vi "quantizzatore.vi"(8 "Segnale input":waveform(dbl), 9 "B (# Bits)":dbl, 10 "Vfs":dbl, 11 "Tipo (bipolare = true)":bool) -> (0 "Livelli":dbl[](array[numeric]), 1 "Segnale quantizzato":waveform(dbl), 2 "2^B":dbl, 3 "Q":dbl)   [LabVIEW 2009]
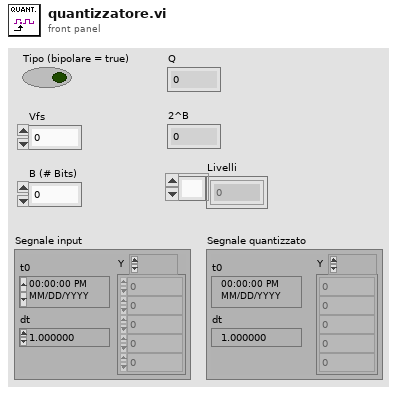
[diagram p1: front panel]
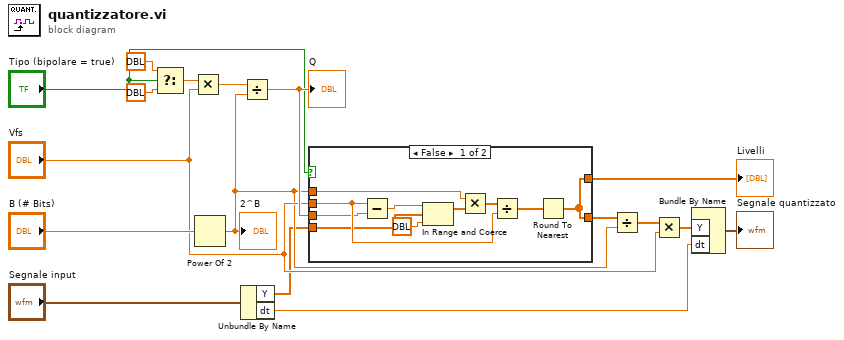
[diagram p0: block diagram]
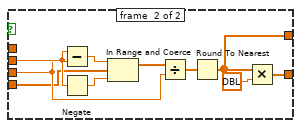
[diagram p2: hidden frame]
diagram:
  n1 = Select(t=dbl ?, s="Tipo (bipolare = true)", f=dbl ?) -> (s? t:f=w13:dbl)
  n2 = Multiply(x=w13, y="Vfs") -> (x*y=w14:dbl)
  n3 = Power Of 2(x="B (# Bits)") -> (2^x=w8:dbl)
  "2^B" <- w8
  n4 = Unbundle By Name("Segnale input") -> ("Y"=w6:dbl[], "dt"=w4:dbl)
  n5 = Divide(x=w14, y=w8) -> (x/y=w17:dbl)
  "Q" <- w17
  n6 = case shown="False" "Tipo (bipolare = true)" {
    tunnel: w6 -> [w24 w32]
    tunnel: [w18 w28] -> w2
    tunnel: "Vfs" -> [w27 w37]
    tunnel: w8 -> [w21 _]
    tunnel: w17 -> [w26 w36]
    tunnel: [w18 w30] -> w1
    frame #0 {
      n7 = Subtract(x=w27, y=w26) -> (x-y=w23:dbl)
      n8 = In Range and Coerce(upper limit=w23, x=w24, lower limit=dbl ?) -> (coerced(x)=w22:dbl[])  [unwired: 1 out]
      n9 = Multiply(x=w21, y=w22) -> (x*y=w20:dbl[])
      n10 = Divide(x=w20, y=w27) -> (x/y=w19:dbl[])
      n11 = Round To Nearest(number=w19) -> (nearest integer value=w18:dbl[])
    }
    frame #1 {
      n12 = Subtract(x=w37, y=w36) -> (x-y=w31:dbl)
      n13 = Negate(x=w37) -> (-x=w33:dbl)
      n14 = In Range and Coerce(upper limit=w31, x=w32, lower limit=w33) -> (coerced(x)=w34:dbl[])  [unwired: 1 out]
      n15 = Divide(x=w34, y=w36) -> (x/y=w35:dbl[])
      n16 = Round To Nearest(number=w35) -> (nearest integer value=w30:dbl[])
      n17 = Multiply(x=w30, y=dbl ?) -> (x*y=w28:dbl[])
    }
  }
  "Livelli" <- w1
  n18 = Divide(x=w2, y=w8) -> (x/y=w16:dbl[])
  n19 = Multiply(x=w16, y="Vfs") -> (x*y=w5:dbl[])
  n20 = Bundle By Name("Y"=w5, "dt"=w4) -> (→"Segnale quantizzato":waveform(dbl))  [unwired: 1 in]
